vi "Read Logging Enabled.vi"(8 "error in (no error)":errorcluster, 11 "Rename in":refnum<class "Rename.lvclass">) -> (0 "error out":errorcluster, 2 "Logging Enabled":bool, 3 "Rename out":refnum<class "Rename.lvclass">)   [LabVIEW 2015, in "Generic Module Library.lvlib" / "Template G_Module.lvlib" / "Rename.lvclass"]
uses:
  Rename.lvclass
  Rename.lvclass/Rename.ctl
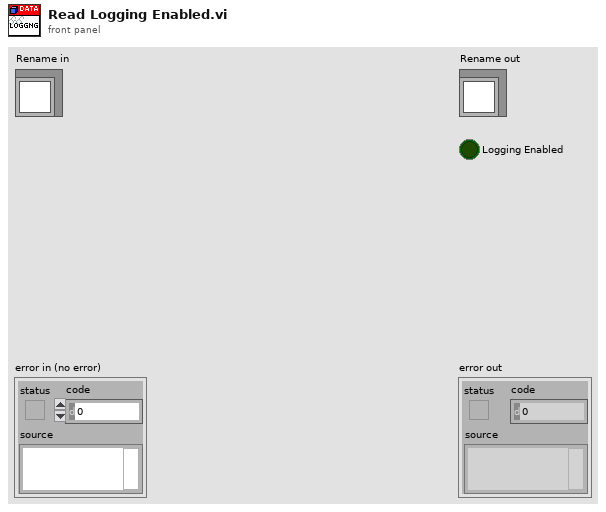
[diagram p1: front panel]
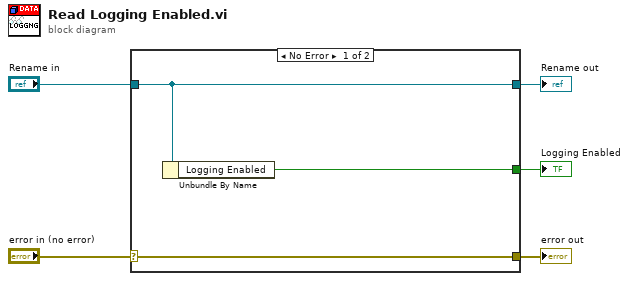
[diagram p0: block diagram]
diagram:
  n1 = case shown="No Error" "error in (no error)" {
    selector: "error in (no error)" -> [w8 w9]
    tunnel: [w8 w9] -> w4
    tunnel: [w7 w10] -> w2
    tunnel: "Rename in" -> [w7 w10]
    tunnel: [w6 _] -> w1
    frame No Error {
      n2 = Unbundle By Name(w7) -> ("Logging Enabled"=w6:bool)
    }
    frame Error {
    }
  }
  "error out" <- w4
  "Rename out" <- w2
  "Logging Enabled" <- w1
